vi "InitializeManager.vi"(8 "error in (no error)":errorcluster, 10 "Path to JSON sequence file":path, 11 "SequenceManager in":refnum<class "SequenceManager.lvclass">) -> (0 "error out":errorcluster, 3 "SequenceManager out":refnum<class "SequenceManager.lvclass">)   [LabVIEW 2023, in "Easy.SequenceManagerLabVIEW.lvlib" / "SequenceManager.lvclass"]
uses:
  SequenceManager.lvclass
  SequenceManager.lvclass/SequenceManager.ctl
  C:/Projects/Cutiss/SequenceManager/SequenceManager/LabViewWrapper/build/Easy.SequenceManager.dll
  build/Easy.SequenceManager.dll
panel:
  # "Connector Pane"
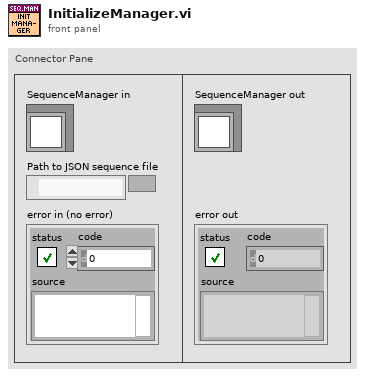
[diagram p1: front panel]
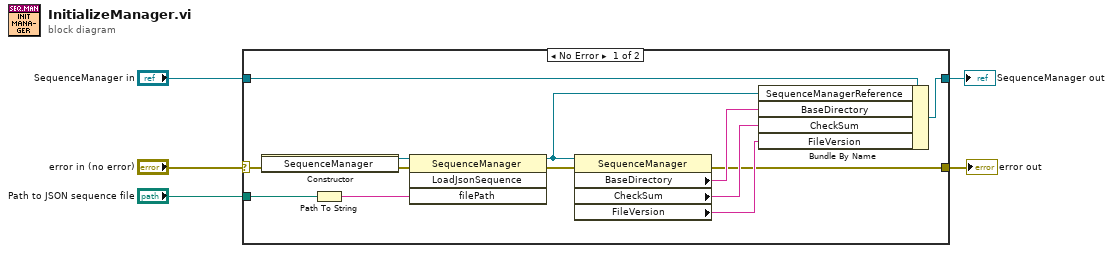
[diagram p0: block diagram]
diagram:
  n1 = case shown="No Error" "error in (no error)" {
    selector: "error in (no error)" -> [w14 w20]
    tunnel: [w6 w20] -> w4
    tunnel: [w13 w19] -> w2
    tunnel: "SequenceManager in" -> [w18 w19]
    tunnel: "Path to JSON sequence file" -> [w12 _]
    frame No Error {
      n2 = constructor class="SequenceManager"(error in=w14) -> (reference out=w17:refnum<k24>, error out=w16:errorcluster)  [unwired: 2 in, 1 out]
      n3 = Path To String(path=w12) -> (string=w15:string)
      n4 = invoke class="SequenceManager" method="LoadJsonSequence"(reference=w17, error in=w16, "filePath"=w15) -> (reference out=w10:refnum<k24>, error out=w11:errorcluster)  [unwired: 1 in, 2 out]
      n5 = property class="SequenceManager"(reference=w10, error in=w11) -> (error out=w6:errorcluster, "BaseDirectory"=w9:string, "CheckSum"=w8:string, "FileVersion"=w7:string)  [unwired: 1 out]
      n6 = Bundle By Name(cluster=w18, "SequenceManagerReference"=w10, "BaseDirectory"=w9, "CheckSum"=w8, "FileVersion"=w7) -> (w13:refnum<class "SequenceManager.lvclass">)
    }
    frame Error {
    }
  }
  "error out" <- w4
  "SequenceManager out" <- w2
